vi "Untitled 1.vi"() -> ()   [LabVIEW 2017]
uses:
  <vilib>/Instr/_visa.llb/VISA Configure Serial Port (Instr).vi
panel:
  in  "stop 3":bool
  out "Waveform Chart":dbl(graph)
  out "error out 2":errorcluster
  out "read buffer 2":string
  in  "stop 2":bool
  in  "ekg":refnum<visa-resource-name>
  out "output 2":dbl
  out "String":string
  out "output 1":dbl
  in  "adxl45":refnum<visa-resource-name>
  in  "stop":bool
  out "read buffer":string
  out "error out":errorcluster
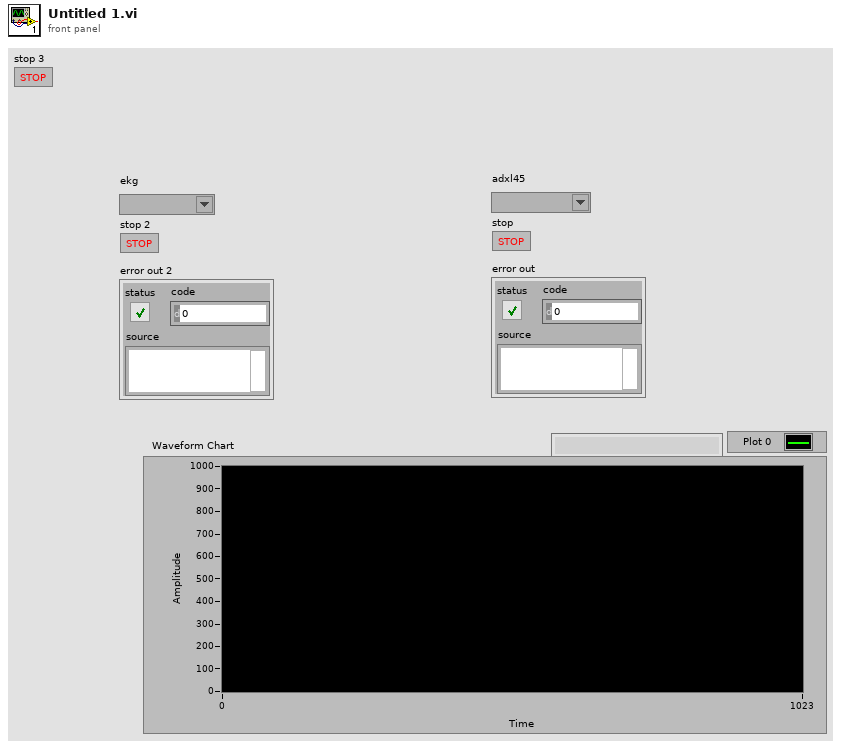
[diagram p1: front panel]
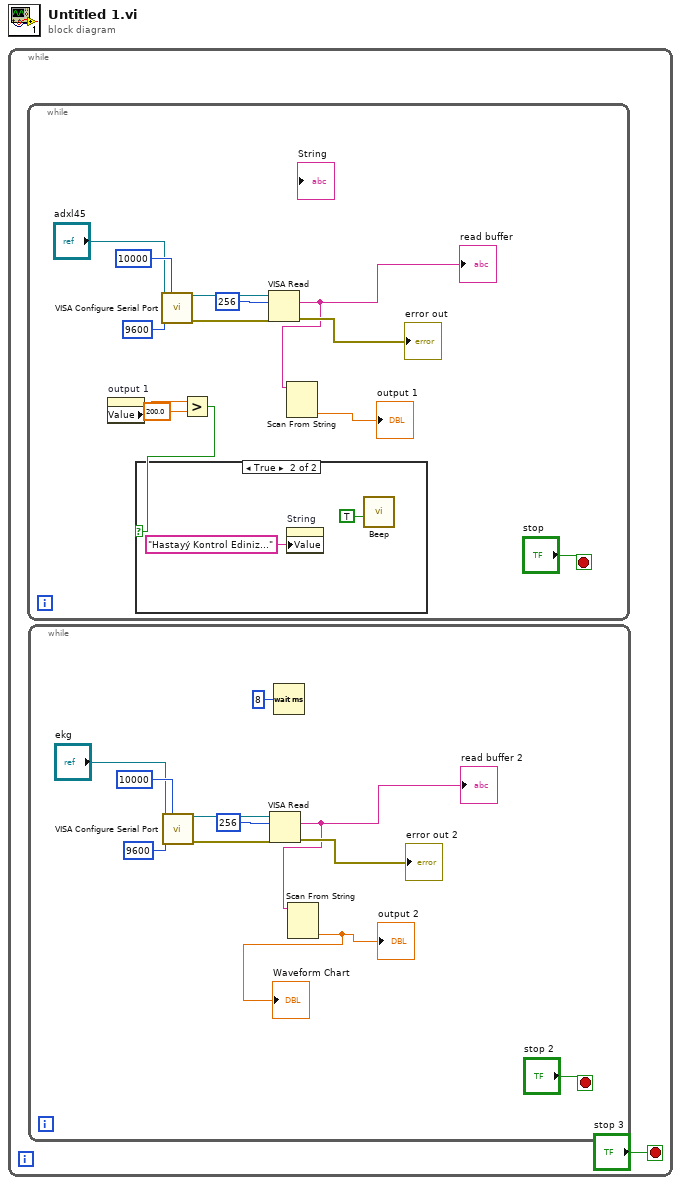
[diagram p0: block diagram]
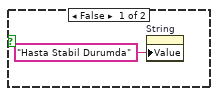
[diagram p2: hidden frame]
diagram:
  n1 = while {
    stop <- "stop 3" stop-if-true
    n2 = while {
      stop <- "stop" stop-if-true
      n3 = property on="output 1" class="DigNum (strict)"() -> ("Value"=w15:dbl)  [unwired: 2 in, 2 out]
      n4 = call-poly "VISA Configure Serial Port"("VISA resource name"="adxl45", "timeout (10sec)"=u32 10000, "baud rate (9600)"=u32 9600) -> ("VISA resource name out"=w23:refnum<visa-resource-name>, "error out"=w22:errorcluster)  [unwired: 11 in]
      n5 = Greater?(x=w15, y=200.0) -> (0:w13:bool)
      n6 = case shown="True" w13 {
        frame False {
          n7 = property on="String" class="Str"("Value"="Hasta Stabil Durumda" ("String")) -> ()  [unwired: 2 in, 2 out]
        }
        frame True {
          n8 = property on="String" class="Str"("Value"="Hastayý Kontrol Ediniz..." ("String")) -> ()  [unwired: 2 in, 2 out]
          n9 = call <vilib>:"Beep.vi"("use system alert? (T)"=TRUE) -> ()  [unwired: 11 in]
        }
      }
      n10 = VISA Read(VISA resource name=w23, byte count=u32 256, error in (no error)=w22) -> (read buffer=w17:string, error out=→"error out":errorcluster)  [unwired: 2 out]
      "read buffer" <- w17
      n11 = Scan From String(input string=w17) -> (output 1=→"output 1":dbl)  [unwired: 4 in, 3 out]
    }
    n12 = while {
      stop <- "stop 2" stop-if-true
      n13 = call-poly "VISA Configure Serial Port"("VISA resource name"="ekg", "timeout (10sec)"=u32 10000, "baud rate (9600)"=u32 9600) -> ("VISA resource name out"=w10:refnum<visa-resource-name>, "error out"=w9:errorcluster)  [unwired: 11 in]
      n14 = VISA Read(VISA resource name=w10, byte count=u32 256, error in (no error)=w9) -> (read buffer=w4:string, error out=→"error out 2":errorcluster)  [unwired: 2 out]
      "read buffer 2" <- w4
      n15 = Wait (ms)(milliseconds to wait=u32 8) -> ()  [unwired: 1 out]
      n16 = Scan From String(input string=w4) -> (output 1=→"output 2" →"Waveform Chart":dbl)  [unwired: 4 in, 3 out]
    }
  }
